vi "Do.vi"(8 "error in":errorcluster, 10 "Actor in":refnum<class "Actor.lvclass">, 11 "Update Device Setpoint MSG":refnum<class "Update Device Setpoint MSG.lvclass">) -> (0 "error out":errorcluster, 2 "Actor out":refnum<class "Actor.lvclass">)   [LabVIEW 2017, in "DAQ Device.lvlib" / "Update Device Setpoint MSG.lvclass"]
doc: "(<B>Filename</B>: Actor Framework.lvlib:Message.lvclass:Do.vi)\n\nDefines what a message does when it is received by an actor. Generally, a message instructs an actor to invoke one of its methods. By default, this method does nothing. A child class must override it to define behavior. Create a child class by using the Actor Framework Message Maker dialog box."
uses:
  Update Device Setpoint MSG.lvclass
  <vilib>/ActorFramework/Actor/Actor.lvclass
  Update Device Setpoint MSG.lvclass/Update Device Setpoint MSG.ctl
  <vilib>/MSR Consulting, LLC/Devices/DAQ Device/Device/Device.lvclass
  C:/Program Files (x86)/National Instruments/LabVIEW 2017/vi.lib/MSR Consulting, LLC/General Reuse/SuperActor/SuperActor.lvclass
  C:/Program Files (x86)/National Instruments/LabVIEW 2017/vi.lib/ActorFramework/Actor/Actor.lvclass
  <vilib>/MSR Consulting, LLC/Devices/DAQ Device/Device/Device.lvclass/Device.ctl
  <vilib>/MSR Consulting, LLC/General Reuse/SuperActor/SuperActor.lvclass/SuperActor.ctl
  <vilib>/MSR Consulting, LLC/Devices/DAQ Device/Device/Read Configurable Device.vi
  <vilib>/MSR Consulting, LLC/General Reuse/SuperActor/Read CVT Session.vi
  <vilib>/MSR Consulting, LLC/General Reuse/SuperActor/Read ID.vi
  <vilib>/MSR Consulting, LLC/General Reuse/Session APIs/_Session Fwk/Session - Root.lvclass
  <vilib>/MSR Consulting, LLC/Devices/Configurable Device/Configurable Device.lvclass
  <vilib>/MSR Consulting, LLC/General Reuse/Session APIs/CVT/CVT.lvclass
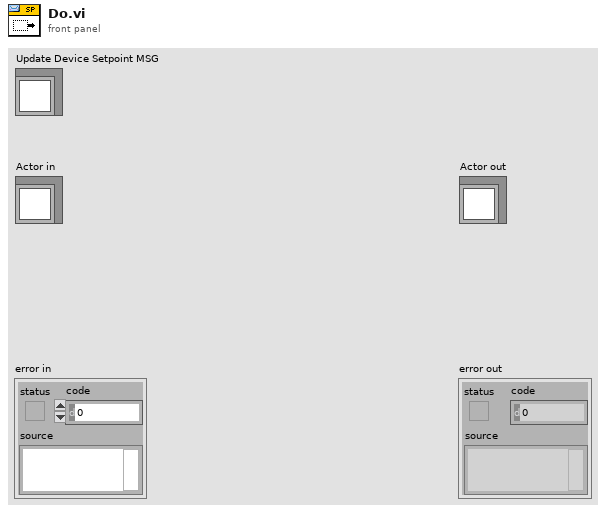
[diagram p1: front panel]
types:
  T1 = typedef "Session - Root.lvclass/Session Handle.ctl" = refnum<data-value>
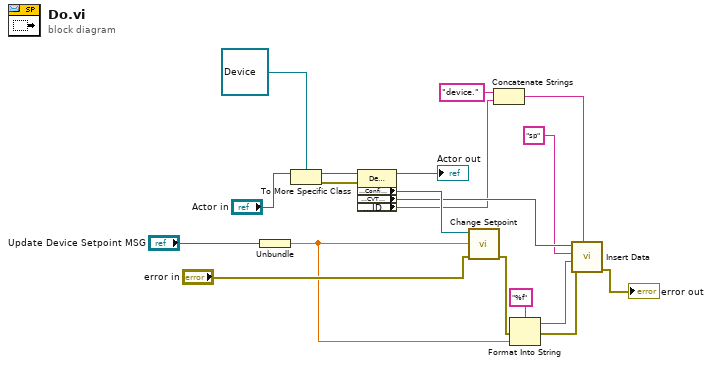
[diagram p0: block diagram]
diagram:
  n1 = Unbundle("Update Device Setpoint MSG") -> (w5:dbl)
  n2 = To More Specific Class(target class=refnum<class "Device.lvclass"> refnum ("DAQ Device.lvlib:Device"), reference="Actor in") -> (specific class reference=w17:refnum<class "Device.lvclass">, error out=w16:errorcluster)  [unwired: 1 in]
  n3 = property class="Device"(reference=w17, error in=w16) -> (reference out=→"Actor out":refnum<class "Device.lvclass">, "Accessors:Configurable Device"=w15:refnum<class "Configurable Device.lvclass">, "Accessors:CVT Session"=w11:T1, "Accessors:ID"=w7:string)  [unwired: 1 out]
  n4 = call-dynamic "Change Setpoint.vi"("error in"="error in", "Setpoint"=w5, "Configurable Device in"=w15) -> ("error out"=w2:errorcluster)  [unwired: 7 in, 1 out]
  n5 = Concatenate Strings("device." ("string"), w7) -> (w6:string)
  n6 = Format Into String(format string="%f", error in=w2, w5) -> (resulting string=w3:string, error out=w1:errorcluster)  [unwired: 1 in]
  n7 = call <vilib>:"Insert Data.vi"("Group"=w6, "error in"=w1, "Data"=w3, "tag"="sp", "CVT Session In"=w11) -> ("error out"=→"error out":errorcluster)  [unwired: 5 in, 1 out]
